vi "Repeat Until Count.vi"(7 "Name":string="Repeat Until Timeout", 8 "On Count Status":T1, 9 "Count":i32, 10 "Finish On":T2, 11 "Node In":refnum<class "abs_Node.lvclass">) -> (3 "Node Out":refnum<class "abs_Node.lvclass">)   [LabVIEW 2021, in "BT.lvlib"]
uses:
  BT.lvlib
  Support/abs_Node/abs_Node.lvclass
  Support/Repeater/Support/Finish On - Type.ctl
  Support/Repeat Until Count/Support/On Count Status - Type.ctl
  Support/Repeat Until Count/Repeat Until Count.lvclass
  C:/Users/Tim/Documents/GitHub/LV_Abstract/Source/Abs_Types/Type/Abs_Type.lvclass
  C:/Users/Tim/Documents/GitHub/LV_Behaviour_Tree/Source/Support/abs_Decorator/abs_Decorator.lvclass
  C:/Users/Tim/Documents/GitHub/LV_Behaviour_Tree/Source/Support/Repeater/Repeater.lvclass
  C:/Users/Tim/Documents/GitHub/LV_Behaviour_Tree/Source/Support/abs_Node/abs_Node.lvclass
  LV_Abstract/Source/Abs_Types/Type/Abs_Type.lvclass/Abs_Type.ctl
  Support/abs_Decorator/abs_Decorator.lvclass/abs_Decorator.ctl
  Support/Repeater/Repeater.lvclass/Repeater.ctl
  Support/Repeat Until Count/Repeat Until Count.lvclass/Repeat Until Count.ctl
  LV_Abstract/Source/Abs_Types/Type/Properties/Write Name.vi
  Support/abs_Decorator/Properties/Write Node.vi
  Support/Repeater/Properties/Write Finish On.vi
  Support/Repeat Until Count/Properties/Write On Count Status.vi
  Support/Repeat Until Count/Properties/Write Count.vi
  Support/Repeater/Repeater.lvclass
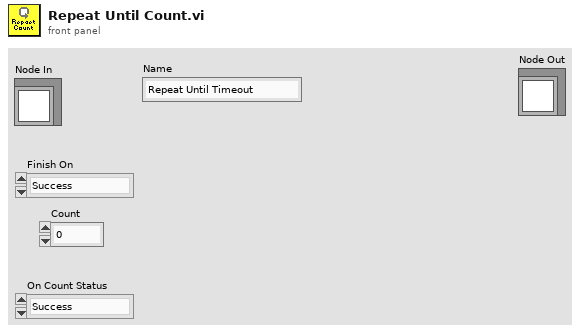
[diagram p1: front panel]
types:
  T1 = typedef "BT.lvlib/Repeat Until Count.lvclass/On Count Status - Type.ctl" = enum16{"Success", "Failure"}
  T2 = typedef "BT.lvlib/Repeater.lvclass/Finish On - Type.ctl" = enum16{"Success", "Failure", "Never"}
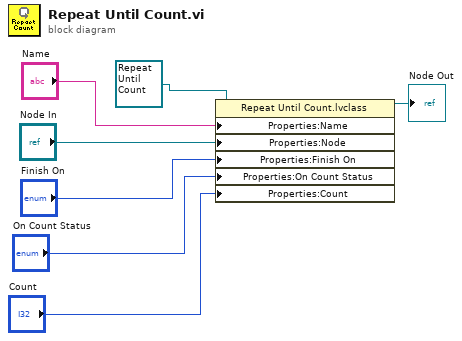
[diagram p0: block diagram]
diagram:
  n1 = property class="Repeat Until Count.lvclass"(reference=refnum<class "Repeat Until Count.lvclass"> refnum ("BT.lvlib:Repeat Until Count.lvclass"), "Properties:Name"="Name", "Properties:Node"="Node In", "Properties:Finish On"="Finish On", "Properties:On Count Status"="On Count Status", "Properties:Count"="Count") -> (reference out=→"Node Out":refnum<class "Repeat Until Count.lvclass">)  [unwired: 1 in, 1 out]
